vi "Q.Enqueue Reset.vi"(4 "Data2":variant, 5 "Top of Q(T)":bool=TRUE, 6 "Data1":variant, 7 "Q Name":string, 8 "Error In":errorcluster, 9 "Sub":string, 10 "Flush Queue(T)":bool=TRUE, 11 "Q In":refnum<queue>) -> (0 "error out":errorcluster, 3 "Q Out":refnum<queue>)   [LabVIEW 2024, in "EQMF.lvlib" / "Queue Utils.lvlib"]
doc: "This VI enqueues the RESET command.\n Queue element 'Cmd' = \"Reset\"\n\nThis VI obtains the queue by name or by queue reference.\nIf the 'Q Name' input is empty then it obtains the queue by the 'Q In\" reference.\nIf the 'Q Name' input is NOT empty then it obtains the queue by the this name.\n If a queue is ontained by name and the queue does not already exits, an error is generated.\n\nThe 'Top of Q' input is TRUE by default.\nThis input will cause this item to be enqueued on the top of the queue when it is TRUE.\n\nThe 'Flush Q' input is TRUE by default.\nThis input will cause the queue to be flushed when it is TRUE."
uses:
  Queue Utils.lvlib
  Q.Element.ctl
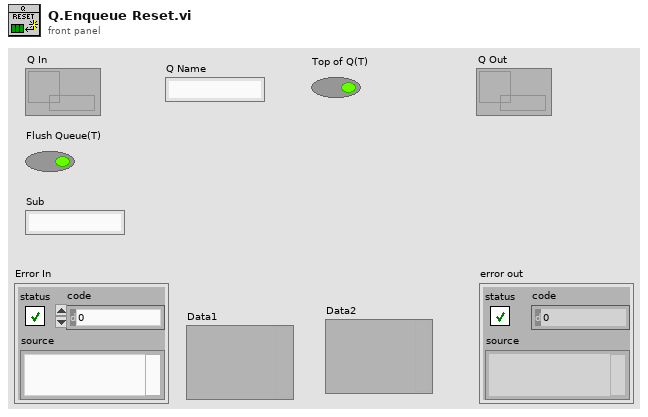
[diagram p1: front panel]
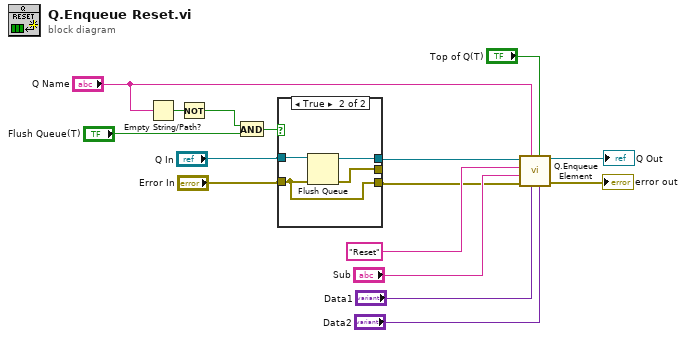
[diagram p0: block diagram]
diagram:
  n1 = Empty String/Path?(string/path="Q Name") -> (empty?=w9:bool)
  n2 = Not(x=w9) -> (.not. x?=w7:bool)
  n3 = And(x=w7, y="Flush Queue(T)") -> (x .and. y?=w8:bool)
  n4 = case shown="True" w8 {
    tunnel: "Q In" -> [w18 w22]
    tunnel: "Error In" -> [w17 w20]
    tunnel: [w18 w21] -> w5
    tunnel: [w17 w20] -> w6
    tunnel: [_ w19] -> _
    frame False {
    }
    frame True {
      n5 = Flush Queue(queue=w22, error in (no error)=w20) -> (queue out=w21:refnum<queue>, error out=w19:errorcluster)  [unwired: 1 out]
    }
  }
  n6 = call "Q.Enqueue Element.vi"("Data2"="Data2", "Top of Q"="Top of Q(T)", "Data1"="Data1", "Q Name"="Q Name", "error in"=w6, "Sub"="Sub", "Cmd"="Reset", "Q In"=w5) -> ("error out"=→"error out":errorcluster, "Q Out"=→"Q Out":refnum<queue>)  [unwired: 2 in]
